vi "NF WF1973_74 BURS Ost.vi"(5 "Type(Half)":bool, 6 "Read(F)":bool, 7 "Mode(Gate)":bool, 8 "error in (no error)":errorcluster caption="Error IN", 10 "Ch(Ch1)":bool, 11 "VISAsession":refnum<visa-resource-name>) -> (0 "error out":errorcluster caption="Error OUT", 2 "Query Mode":string, 3 "CopyVISAsession":refnum<visa-resource-name>)   [LabVIEW 2010]
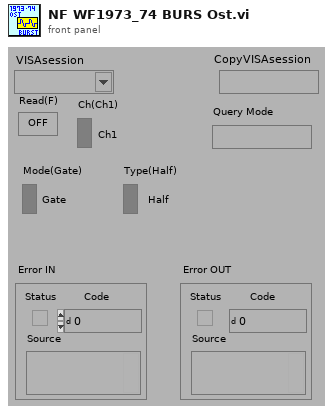
[diagram p1: front panel]
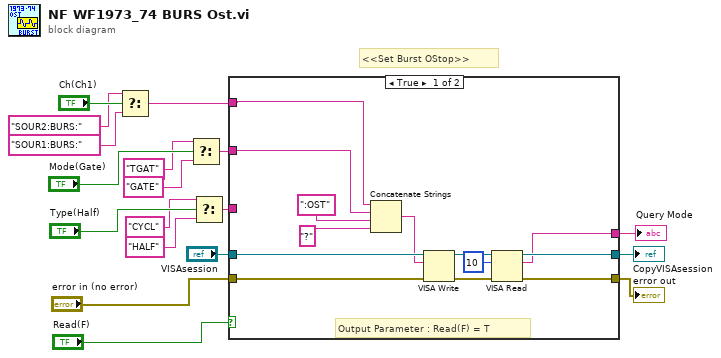
[diagram p0: block diagram]
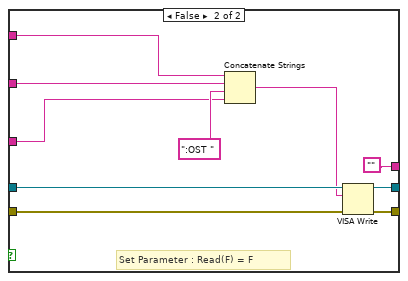
[diagram p2: hidden frame]
diagram:
  # "<<Set Burst OStop>>"
  n1 = Select(t="SOUR2:BURS:" ("文字列"), s="Ch(Ch1)", f="SOUR1:BURS:" ("文字列")) -> (s? t:f=w11:string)
  n2 = Select(t="TGAT", s="Mode(Gate)", f="GATE") -> (s? t:f=w5:string)
  n3 = Select(t="CYCL", s="Type(Half)", f="HALF") -> (s? t:f=w1:string)
  n4 = case shown="TRUE" "Read(F)" {
    tunnel: "VISAsession" -> [w31 w41]
    tunnel: [w28 w39] -> w17
    tunnel: [w27 w40] -> w16
    tunnel: "error in (no error)" -> [w26 w36]
    tunnel: w11 -> [w22 w37]
    tunnel: [w23 ""] -> w13
    tunnel: w5 -> [w21 w34]
    tunnel: w1 -> [_ w32]
    frame True {
      # "Output Parameter : Read(F) = T"
      n5 = Concatenate Strings(w22, w21, ":OST" ("形式文字列"), "?" ("形式文字列")) -> (w24:string)
      n6 = VISA Write(VISA resource name=w31, write buffer=w24, error in (no error)=w26) -> (VISA resource name out=w29:refnum<visa-resource-name>, error out=w30:errorcluster)  [unwired: 1 out]
      n7 = VISA Read(VISA resource name=w29, byte count=u32 10 ("バイトカウント（0）"), error in (no error)=w30) -> (VISA resource name out=w28:refnum<visa-resource-name>, read buffer=w23:string, error out=w27:errorcluster)  [unwired: 1 out]
    }
    frame False {
      # "Set Parameter : Read(F) = F"
      n8 = Concatenate Strings(w37, w34, ":OST " ("文字列"), w32) -> (w38:string)
      n9 = VISA Write(VISA resource name=w41, write buffer=w38, error in (no error)=w36) -> (VISA resource name out=w39:refnum<visa-resource-name>, error out=w40:errorcluster)  [unwired: 1 out]
    }
  }
  "error out" <- w16
  "CopyVISAsession" <- w17
  "Query Mode" <- w13
